vi "周期设置_总氮.vi"() -> ()   [LabVIEW 2016, in "斯坦道总氮.lvlib"]
uses:
  <vilib>/Utility/miscctls.llb/LVPointTypeDef.ctl
  <vilib>/Utility/config.llb/NI_LVConfig.lvlib
panel:
  in  "运行周期":T1={"运行模式"=enum."维护模式", "质控频次"=enum."关闭", "空白核查时间"=2, "跨度核查时间"=6, "24H周期设置"=[]} {"跨度核查时间" items=["00H", "01H", "02H", "03H", "04H", "05H", "06H", "07H", "08H", "09H", "10H", "11H", "12H", "13H", "14H", "15H", "16H", "17H", "18H", "19H", "20H", "21H", "22H", "23H", "关闭"]; "空白核查时间" items=["00H", "01H", "02H", "03H", "04H", "05H", "06H", "07H", "08H", "09H", "10H", "11H", "12H", "13H", "14H", "15H", "16H", "17H", "18H", "19H", "20H", "21H", "22H", "23H", "关闭"]}
  # "运行模式："
  # "质控频次："
  # "零点核查时间："
  # "跨度核查时间："
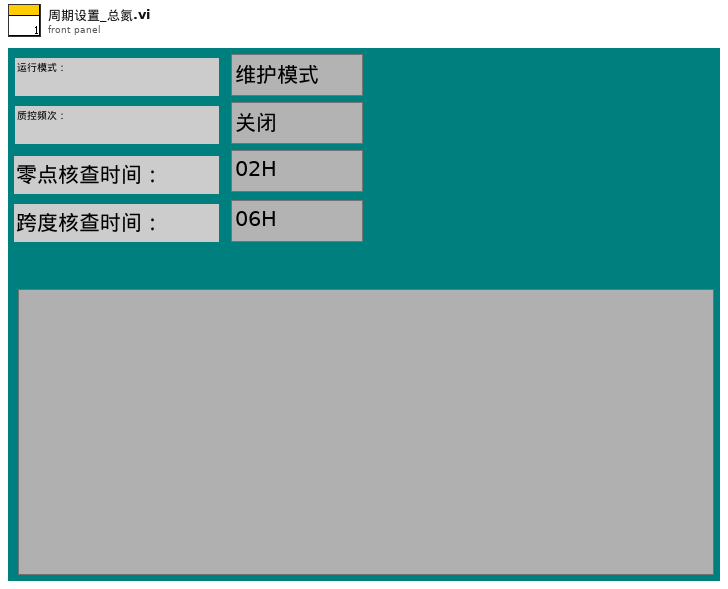
[diagram p1: front panel]
types:
  T1 = cluster{"运行模式":enum16{"维护模式", "常规模式", "应急模式", "质控模式"}, "质控频次":enum16{"关闭", "每天", "星期一", "星期二", "星期三", "星期四", "星期五", "星期六", "星期日"}, "空白核查时间":u16, "跨度核查时间":u16, "24H周期设置":bool[]}
  T2 = typedef "LVPointTypeDef.ctl" = cluster{"Horizontal":i16, "Vertical":i16}
  T3 = enum16{"启动测量", "标样核查", "零点核查", "跨度核查", "空白测试", "平行样测试", "加标回收", "空白校准", "标样校准", "初始化（清洗）", "停止测试", "仪器重启", "校时", "模式设置", "测量间隔设置"}
  T4 = enum16{"关闭", "每天", "星期一", "星期二", "星期三", "星期四", "星期五", "星期六", "星期日"}
  T5 = typedef "LVDateTimeRec.ctl" = cluster{"秒数的小数部分":dbl, "秒":i32, "分":i32, "时":i32, "日":i32, "月":i32, "年":i32, "天数（周）":i32, "天数（年）":i32, "DST":i32}
  T6 = enum32{"Bad", "Idle", "Run top level", "Running"}
  T7 = typedef "NI_LVConfig.lvlib/Config Data RefNum.ctl" = refnum<k1>
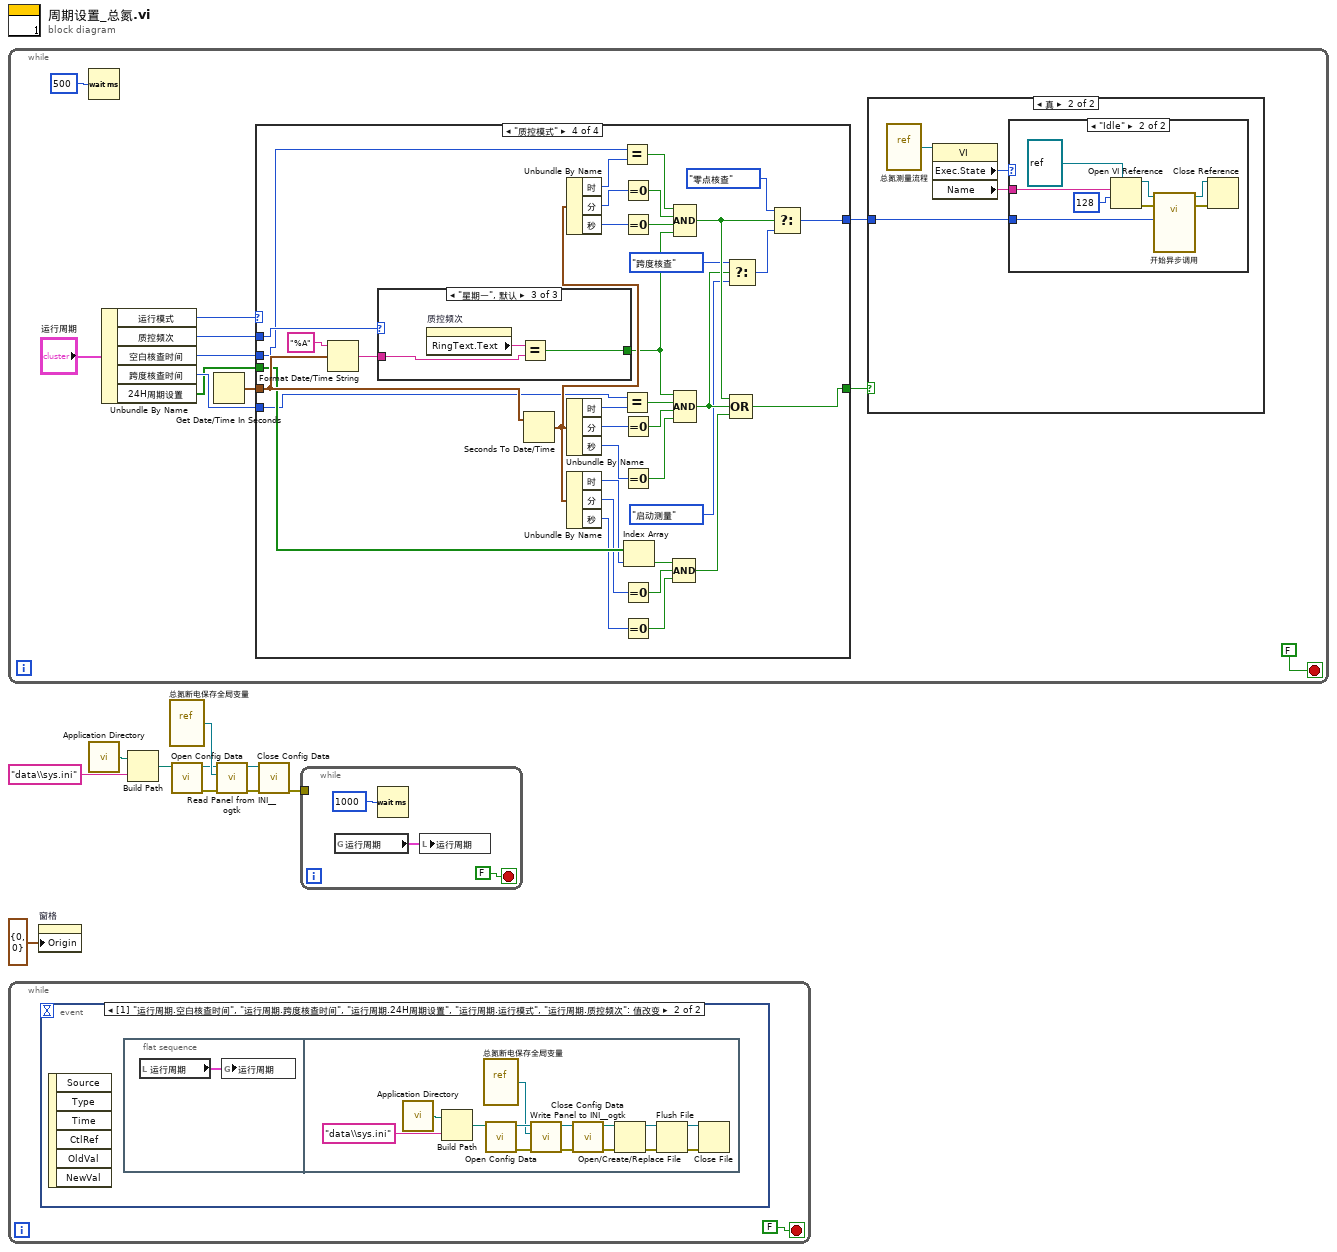
[diagram p0: block diagram]
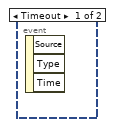
[diagram p2: hidden frame]
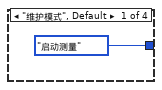
[diagram p5: hidden frame]
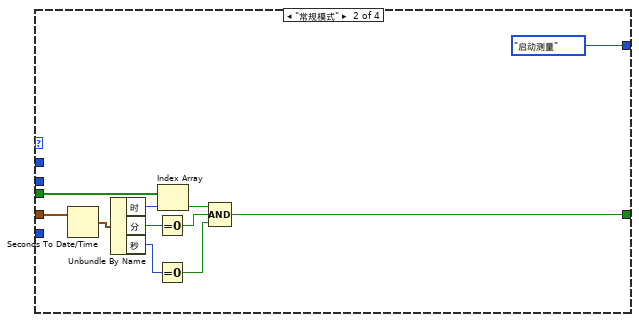
[diagram p6: hidden frame]
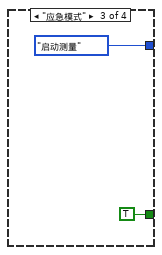
[diagram p7: hidden frame]
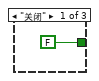
[diagram p8: hidden frame]
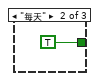
[diagram p9: hidden frame]
diagram:
  n1 = while {
    stop <- FALSE stop-if-true
    n2 = Wait (ms)(milliseconds to wait=u32 500 ("等待时间（毫秒）")) -> ()  [unwired: 1 out]
    n3 = Unbundle By Name("运行周期") -> ("运行模式"=w17:enum16{"维护模式", "常规模式", "应急模式", "质控模式"}, "质控频次"=w16:T4, "空白核查时间"=w15:u16, "跨度核查时间"=w14:u16, "24H周期设置"=w13:bool[])
    n4 = Get Date/Time In Seconds() -> (seconds since 1Jan1904=w21:timestamp)
    n5 = case shown="\"质控模式\"" w17 {
      tunnel: w21 -> [_ w45 _ w83]
      tunnel: w13 -> [_ w42 _ w80]
      tunnel: [_ w36 TRUE w60] -> w12
      tunnel: [T3."启动测量" ("控制命令") T3."启动测量" ("控制命令") T3."启动测量" ("控制命令") w56] -> w11
      tunnel: w16 -> [_ _ _ w53]
      tunnel: w15 -> [_ _ _ w52]
      tunnel: w14 -> [_ _ _ w51]
      frame "维护模式", Default {
      }
      frame "常规模式" {
        n6 = Seconds To Date/Time(time stamp (now)=w45) -> (date time rec=w44:T5)  [unwired: 1 in]
        n7 = Unbundle By Name(w44) -> ("时"=w43:i32, "分"=w41:i32, "秒"=w40:i32)
        n8 = Equal To 0?(x=w41) -> (x = 0?=w38:bool)
        n9 = Equal To 0?(x=w40) -> (x = 0?=w37:bool)
        n10 = Index Array(array=w42, index=w43) -> (element=w39:bool)
        n11 = Compound Arithmetic op=AND ("复合运算")(w39, w38, w37) -> (w36:bool)
      }
      frame "应急模式" {
      }
      frame "质控模式" {
        n12 = Format Date/Time String(time format string (%c)="%A" ("时间格式字符串(%c)"), seconds (now)=w83) -> (date/time string=w81:string)  [unwired: 1 in]
        n13 = case shown="\"星期一\", 默认" w53 {
          tunnel: w81 -> [_ _ w87]
          tunnel: [FALSE TRUE w86] -> w54
          frame "关闭" {
          }
          frame "每天" {
          }
          frame "星期一", Default {
            n14 = property on="质控频次" class="Enum (严格)"() -> ("RingText.Text"=w88:string)  [unwired: 2 in, 2 out]
            n15 = Equal?(x=w88, y=w87) -> (x = y?=w86:bool)
          }
        }
        n16 = Seconds To Date/Time(time stamp (now)=w83) -> (date time rec=w64:T5)  [unwired: 1 in]
        n17 = Unbundle By Name(w64) -> ("时"=w73:i32, "分"=w72:i32, "秒"=w71:i32)
        n18 = Unbundle By Name(w64) -> ("时"=w65:i32, "分"=w66:i32, "秒"=w67:i32)
        n19 = Unbundle By Name(w64) -> ("时"=w79:i32, "分"=w77:i32, "秒"=w75:i32)
        n20 = Equal?(x=w52, y=w73) -> (x = y?=w70:bool)
        n21 = Equal?(x=w51, y=w65) -> (x = y?=w63:bool)
        n22 = Equal To 0?(x=w72) -> (x = 0?=w69:bool)
        n23 = Equal To 0?(x=w71) -> (x = 0?=w68:bool)
        n24 = Equal To 0?(x=w66) -> (x = 0?=w62:bool)
        n25 = Equal To 0?(x=w67) -> (x = 0?=w61:bool)
        n26 = Equal To 0?(x=w77) -> (x = 0?=w76:bool)
        n27 = Equal To 0?(x=w75) -> (x = 0?=w74:bool)
        n28 = Index Array(array=w80, index=w79) -> (element=w78:bool)
        n29 = Compound Arithmetic op=AND ("复合运算")(w78, w76, w74) -> (w55:bool)
        n30 = Compound Arithmetic op=AND ("复合运算")(w70, w69, w68, w54) -> (w59:bool)
        n31 = Compound Arithmetic op=AND ("复合运算")(w54, w63, w62, w61) -> (w58:bool)
        n32 = Select(t=T3."跨度核查" ("控制命令"), s=w58, f=T3."启动测量" ("控制命令")) -> (s? t:f=w57:T3)
        n33 = Compound Arithmetic op=OR ("复合运算")(w59, w58, w55) -> (w60:bool)
        n34 = Select(t=T3."零点核查" ("控制命令"), s=w59, f=w57) -> (s? t:f=w56:T3)
      }
    }
    n35 = case shown="真" w12 {
      tunnel: w11 -> [_ w23]
      frame False {
      }
      frame True {
        n36 = vi-ref "总氮测量流程.vi"() -> (w24:refnum<vi>)
        n37 = property class="VI"(reference=w24) -> ("Exec.State"=w22:T6, "Name"=w25:string)  [unwired: 1 in, 2 out]
        n38 = case shown="\"Idle\"" w22 {
          tunnel: w25 -> [_ w29]
          tunnel: w23 -> [_ w27]
          frame "Bad", Default {
          }
          frame "Idle" {
            n39 = Open VI Reference(type specifier VI Refnum (for type only)=refnum<vi> refnum, vi path=w29, options=128 ("选项")) -> (vi reference=w30:refnum<vi>, error out=w31:errorcluster)  [unwired: 3 in]
            n40 = call-by-ref "开始异步调用"(reference=w30, error in=w31, "控制命令"=w27) -> (reference out=w32:refnum<vi>, error out=w33:errorcluster)  [unwired: 11 in]
            n41 = Close Reference(reference=w32, error in (no error)=w33) -> ()  [unwired: 1 out]
          }
        }
      }
    }
  }
  n42 = while {
    stop <- FALSE stop-if-true
    n43 = event shown="[1] \"运行周期.空白核查时间\", \"运行周期.跨度核查时间\", \"运行周期.24H周期设置\", \"运行周期.运行模式\", \"运行周期.质控频次\": 值改变" {
      selector: _ -> [_ _]
      dyn-events: _ -> [_ _]
      timeout: _ -> [_ _]
      event Timeout {
        n44 = event-data() -> ()  [unwired: 1 in, 3 out]
      }
      event "运行周期.空白核查时间", "运行周期.跨度核查时间", "运行周期.24H周期设置", "运行周期.运行模式", "运行周期.质控频次": Value Change {
        n45 = event-data() -> ()  [unwired: 1 in, 6 out]
        n46 = flat-sequence {
          frame #0 {
            n47 = local read "运行周期"() -> (w90:T1)
            n48 = global write "总氮断电保存全局变量.vi" "运行周期"(w90) -> ()
          }
          frame #1 {
            n49 = call <vilib>:"Application Directory.vi"() -> ("Application Directory"=w104:path)
            n50 = Build Path(base path=w104, name or relative path="data\\sys.ini" ("名称或相对路径")) -> (appended path=w102:path)
            n51 = vi-ref "总氮断电保存全局变量.vi"() -> (w100:refnum<vi>)
            n52 = call <vilib>:"Open Config Data.vi"("configuration file path"=w102) -> ("error out"=w98:errorcluster, "refnum"=w101:T7)  [unwired: 8 in, 1 out]
            n53 = call <userlib>:"Write Panel to INI__ogtk.vi"("error in (no error)"=w98, "VI ref"=w100, "refnum"=w101) -> ("error out"=w97:errorcluster, "refnum out"=w99:T7)  [unwired: 7 in]
            n54 = call <vilib>:"Close Config Data.vi"("error in (no error)"=w97, "refnum"=w99) -> ("error out"=w92:errorcluster, "file path"=w91:path)  [unwired: 8 in]
            n55 = Open/Create/Replace File(file path (use dialog)=w91, error in=w92) -> (refnum out=w95:refnum<file>, error out=w96:errorcluster)  [unwired: 4 in, 1 out]
            n56 = Flush File(refnum=w95, error in=w96) -> (refnum out=w94:refnum<file>, error out=w93:errorcluster)
            n57 = Close File(refnum=w94, error in=w93) -> ()  [unwired: 2 out]
          }
        }
      }
    }
  }
  n58 = property on="窗格" class="Pane"("Origin"=T2 {"Horizontal"=0, "Vertical"=0} ("原点")) -> ()  [unwired: 2 in, 2 out]
  n59 = call <vilib>:"Application Directory.vi"() -> ("Application Directory"=w3:path)
  n60 = Build Path(base path=w3, name or relative path="data\\sys.ini" ("名称或相对路径")) -> (appended path=w5:path)
  n61 = vi-ref "总氮断电保存全局变量.vi"() -> (w7:refnum<vi>)
  n62 = call <vilib>:"Open Config Data.vi"("configuration file path"=w5) -> ("error out"=w9:errorcluster, "refnum"=w6:T7)  [unwired: 8 in, 1 out]
  n63 = call <userlib>:"Read Panel from INI__ogtk.vi"("error in (no error)"=w9, "VI ref"=w7, "refnum"=w6) -> ("error out"=w10:errorcluster, "refnum out"=w8:T7)  [unwired: 7 in]
  n64 = call <vilib>:"Close Config Data.vi"("error in (no error)"=w10, "refnum"=w8) -> ("error out"=w2:errorcluster)  [unwired: 8 in, 1 out]
  n65 = while {
    tunnel: w2 -> [_]
    stop <- FALSE stop-if-true
    n66 = global read "总氮断电保存全局变量.vi" "运行周期"() -> (w105:T1)
    n67 = Wait (ms)(milliseconds to wait=u32 1000 ("等待时间（毫秒）")) -> ()  [unwired: 1 out]
    n68 = local write "运行周期"(w105) -> ()
  }
